vi "read PointGrey metadata file.vi"(0 "PointGrey metadata file path":path) -> (3 "Frames On File":i32, 4 "Created Csv File":path, 6 "Frame Drops":i64, 8 "Frames Acquired":i32, 10 "FrameCounter (processed)":i64[](array[numeric]), 13 "Separation Character":string, 15 "File Has Data":bool)   [LabVIEW 2010]
uses:
  <vilib>/Utility/file.llb/Read From Spreadsheet File (I64).vi
panel:
  out "Original File Lines":string[](array[string])
  out "Frequency (approximate)":ext format="%#.2g"
  out "PointGrey Timestamp (seconds)":ext[](array[numeric])
  out "TimeStamp (raw)":i64[](array[numeric])
  out "FrameCounter (raw)":i64[](array[numeric])
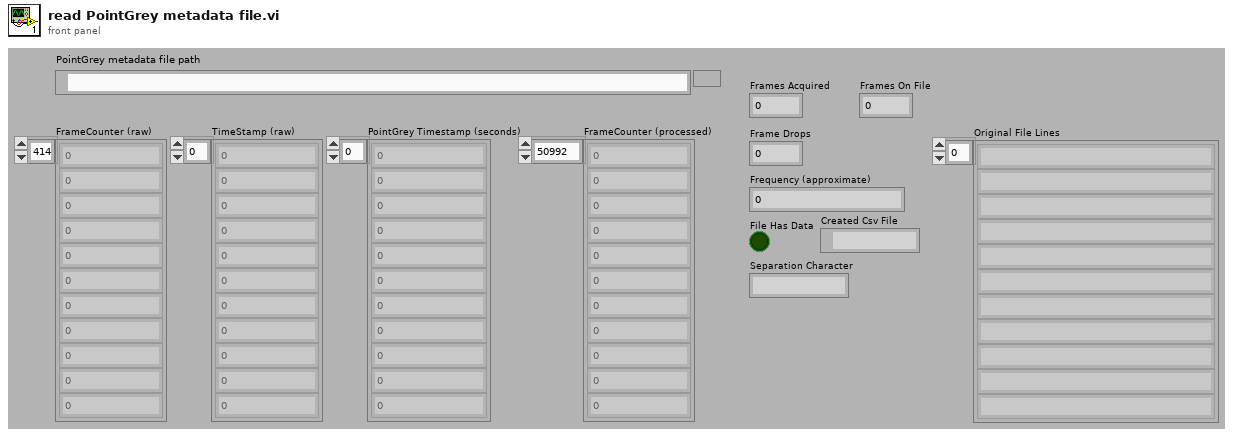
[diagram p1: front panel]
types:
  T1 = enum16{"open", "replace", "create", "open or create", "replace or create", "replace or create with confirmation"}
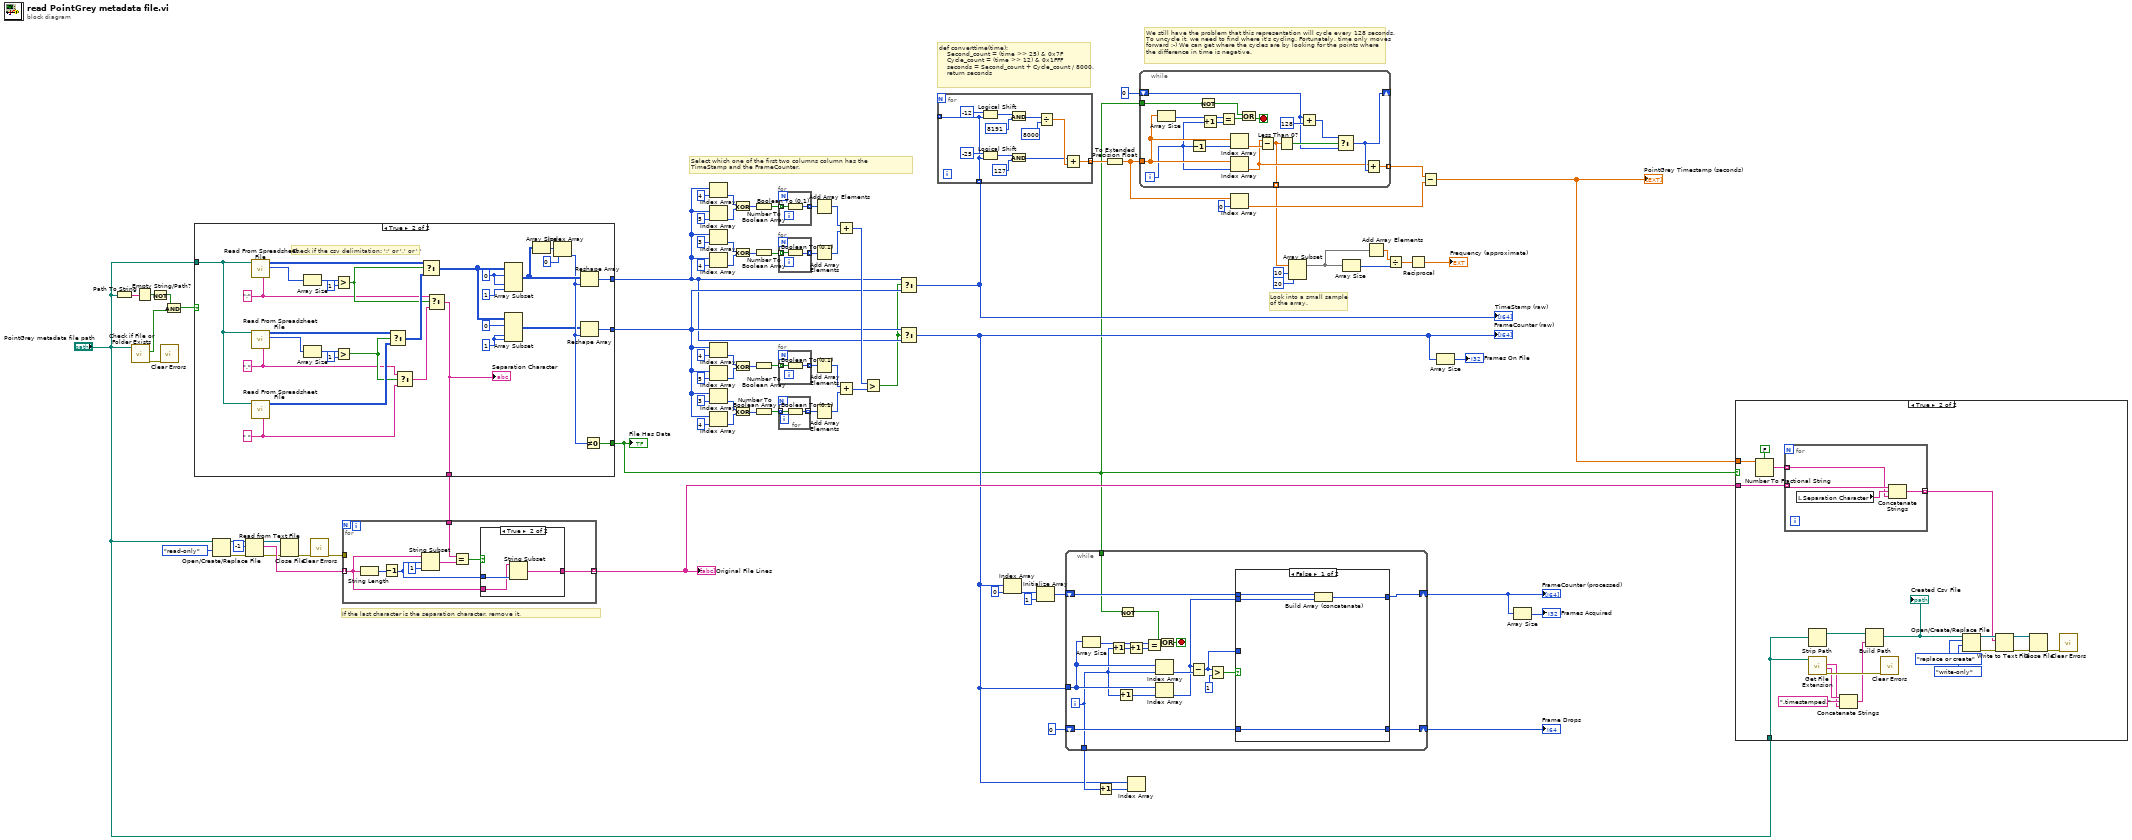
[diagram p0: block diagram]
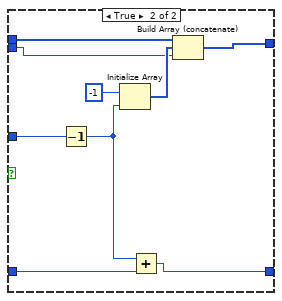
[diagram p4: hidden frame]
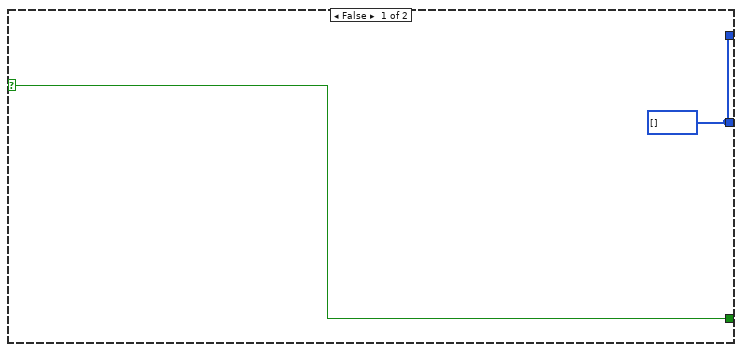
[diagram p5: hidden frame]
diagram:
  # "If the last character is the separation character, remove it."
  # "Select which one of the first two columns column has the\nTimeStamp and the FrameCounter."
  # "Look into a small sample\nof the array."
  # "We still have the problem that this representation will cycle every 128 seconds.\nTo uncycle it, we need to find where it's cycling. Fortunately, time only moves\nforward :-) We can get where the cycles are by looking for the points where\nthe difference in time is negative."
  # "def converttime(time):\n    Second_count = (time >> 25) & 0x7F\n    Cycle_count = (time >> 12) & 0x1FFF\n    seconds = Second_count + Cycle_count / 8000.\n    return seconds"
  n1 = Path To String(path="PointGrey metadata file path") -> (string=w5:string)
  n2 = call <vilib>:"Check if File or Folder Exists.vi"("path"="PointGrey metadata file path") -> ("error out"=w84:errorcluster, "file or folder exists?"=w83:bool)  [unwired: 8 in, 1 out]
  n3 = Empty String/Path?(string/path=w5) -> (empty?=w4:bool)
  n4 = Not(x=w4) -> (.not. x?=w2:bool)
  n5 = call <vilib>:"Clear Errors.vi"("error in (no error)"=w84) -> ()  [unwired: 6 in, 1 out]
  n6 = And(x=w2, y=w83) -> (x .and. y?=w3:bool)
  n7 = case shown="True" w3 {
    selector: w3 -> [w86 _]
    tunnel: "PointGrey metadata file path" -> [_ w108]
    tunnel: [w85 w101] -> w27
    tunnel: [w86 w109] -> w1
    tunnel: [w85 w99] -> w28
    tunnel: [_ w87] -> w16
    frame False {
      w85 = i64[] []
    }
    frame True {
      w89 = 1 ("length")
      w92 = " " ("delimiter (\\t)")
      w90 = 0 ("index")
      w93 = "," ("delimiter (\\t)")
      w95 = ";" ("delimiter (\\t)")
      # "Check if the csv delimitation: ';' or ',' or ' '"
      n8 = call-poly <vilib>:"Read From Spreadsheet File.vi"("delimiter (\\t)"=w95, "file path (dialog if empty)"=w108) -> ("first row"=w115:i64[], "all rows"=w114:i64[][])  [unwired: 5 in, 3 out]
      n9 = call-poly <vilib>:"Read From Spreadsheet File.vi"("delimiter (\\t)"=w93, "file path (dialog if empty)"=w108) -> ("first row"=w105:i64[], "all rows"=w104:i64[][])  [unwired: 5 in, 3 out]
      n10 = call-poly <vilib>:"Read From Spreadsheet File.vi"("delimiter (\\t)"=w92, "file path (dialog if empty)"=w108) -> ("all rows"=w103:i64[][])  [unwired: 5 in, 4 out]
      n11 = Array Size(array=w115) -> (size(s)=w117:i32)
      n12 = Array Size(array=w105) -> (size(s)=w106:i32)
      n13 = Greater?(x=w117, y=1) -> (0:w96:bool)
      n14 = Greater?(x=w106, y=1) -> (0:w94:bool)
      n15 = Select(t=w104, s=w94, f=w103) -> (s? t:f=w102:i64[][])
      n16 = Select(t=w93, s=w94, f=w92) -> (s? t:f=w91:string)
      n17 = Select(t=w114, s=w96, f=w102) -> (s? t:f=w88:i64[][])
      n18 = Select(t=w95, s=w96, f=w91) -> (s? t:f=w87:string)
      "Separation Character" <- w87
      n19 = Array Subset(array=w88, index (row)=w90, index (col)=w90, length (col)=1 ("length")) -> (w110:i64[][])  [unwired: 1 in]
      n20 = Array Subset(array=w88, index (row)=0 ("index"), index (col)=w89, length (col)=w89) -> (w97:i64[][])  [unwired: 1 in]
      n21 = Array Size(array=w110) -> (size(s)=w112:i32[])
      n22 = Index Array(array=w112, index=0) -> (element=w98:i32)
      n23 = Reshape Array(w110, w98) -> (w101:i64[])
      n24 = Reshape Array(w97, w98) -> (w99:i64[])
      n25 = Not Equal To 0?(x=w98) -> (x != 0?=w109:bool)
    }
  }
  "File Has Data" <- w1
  n26 = Open/Create/Replace File(file path (use dialog)="PointGrey metadata file path", access (0:read/write)=enum16{"read/write", "read-only", "write-only"}."read-only") -> (refnum out=w23:refnum<file>, error out=w24:errorcluster)  [unwired: 4 in, 1 out]
  n27 = Read from Text File(file (use dialog)=w23, count=-1, error in=w24) -> (refnum out=w18:refnum<file>, text=w20:string[], error out=w19:errorcluster)  [unwired: 1 in, 1 out]
  n28 = Close File(refnum=w18, error in=w19) -> (error out=w17:errorcluster)  [unwired: 1 out]
  n29 = call <vilib>:"Clear Errors.vi"("error in (no error)"=w17) -> ("error out"=w14:errorcluster)  [unwired: 6 in]
  n30 = for {
    tunnel: w20 -> [w121] mode=indexing
    tunnel: w14 -> [_]
    tunnel: w16 -> [w122]
    tunnel: [w119] -> w12 mode=indexing
    n31 = String Length(string=w121) -> (length=w125:i32)
    n32 = Decrement(x=w125) -> (x-1=w120:i32)
    n33 = String Subset(string=w121, offset (0)=w120, length (rest)=1 ("length (rest)")) -> (substring=w123:string)
    n34 = Equal?(x=w122, y=w123) -> (x = y?=w118:bool)
    n35 = case shown="True" w118 {
      tunnel: w121 -> [w126 w127]
      tunnel: w120 -> [_ w129]
      tunnel: [w126 w128] -> w119
      frame False {
      }
      frame True {
        n36 = String Subset(string=w127, length (rest)=w129) -> (substring=w128:string)  [unwired: 1 in]
      }
    }
  }
  "Original File Lines" <- w12
  n37 = Index Array(array=w27, index=4) -> (element=w45:i64)
  n38 = Index Array(array=w27, index=5) -> (element=w44:i64)
  n39 = Index Array(array=w27, index=3) -> (element=w59:i64)
  n40 = Index Array(array=w27, index=4) -> (element=w60:i64)
  n41 = Index Array(array=w28, index=4) -> (element=w58:i64)
  n42 = Index Array(array=w28, index=5) -> (element=w57:i64)
  n43 = Index Array(array=w28, index=3) -> (element=w36:i64)
  n44 = Index Array(array=w28, index=4) -> (element=w37:i64)
  n45 = Exclusive Or(1:w44, 2:w45) -> (0:w46:i64)
  n46 = Exclusive Or(1:w60, 2:w59) -> (0:w54:i64)
  n47 = Exclusive Or(1:w57, 2:w58) -> (0:w53:i64)
  n48 = Exclusive Or(1:w37, 2:w36) -> (0:w40:i64)
  n49 = Number To Boolean Array(number=w46) -> (Boolean array=w47:bool[])
  n50 = Number To Boolean Array(number=w54) -> (Boolean array=w52:bool[])
  n51 = Number To Boolean Array(number=w53) -> (Boolean array=w49:bool[])
  n52 = Number To Boolean Array(number=w40) -> (Boolean array=w41:bool[])
  n53 = for {
    tunnel: w41 -> [w131] mode=indexing
    tunnel: [w130] -> _ mode=indexing
    tunnel: [w130] -> w15 mode=indexing
    n54 = Boolean To (0,1)(Boolean=w131) -> (0, 1=w130:i16)
  }
  n55 = for {
    tunnel: w47 -> [w133] mode=indexing
    tunnel: [w132] -> w48 mode=indexing
    n56 = Boolean To (0,1)(Boolean=w133) -> (0, 1=w132:i16)
  }
  n57 = for {
    tunnel: w52 -> [w135] mode=indexing
    tunnel: [w134] -> w51 mode=indexing
    n58 = Boolean To (0,1)(Boolean=w135) -> (0, 1=w134:i16)
  }
  n59 = for {
    tunnel: w49 -> [w137] mode=indexing
    tunnel: [w136] -> w50 mode=indexing
    n60 = Boolean To (0,1)(Boolean=w137) -> (0, 1=w136:i16)
  }
  n61 = Add Array Elements(numeric array=w48) -> (sum=w34:i16)
  n62 = Add Array Elements(numeric array=w51) -> (sum=w35:i16)
  n63 = Add Array Elements(numeric array=w50) -> (sum=w33:i16)
  n64 = Add Array Elements(numeric array=w15) -> (sum=w32:i16)
  n65 = Add(x=w34, y=w35) -> (x+y=w30:i16)
  n66 = Add(x=w33, y=w32) -> (x+y=w31:i16)
  n67 = Greater?(x=w30, y=w31) -> (0:w26:bool)
  n68 = Select(t=w27, s=w26, f=w28) -> (s? t:f=w29:i64[])
  "TimeStamp (raw)" <- w29
  n69 = Select(t=w28, s=w26, f=w27) -> (s? t:f=w7:i64[])
  "FrameCounter (raw)" <- w7
  n70 = for {
    tunnel: [w139] -> _ mode=indexing
    tunnel: [w140] -> w82 mode=indexing
    tunnel: w29 -> [w139] mode=indexing
    n71 = Logical Shift(y=i8 -12, x=w139) -> (x << y=w148:i64)
    n72 = Logical Shift(y=i8 -25, x=w139) -> (x << y=w145:i64)
    n73 = And(x=w148, y=i64 8191) -> (x .and. y?=w143:i64)
    n74 = And(x=w145, y=i64 127) -> (x .and. y?=w138:i64)
    n75 = Divide(x=w143, y=i64 8000) -> (x/y=w141:dbl)
    n76 = Add(x=w138, y=w141) -> (x+y=w140:dbl)
  }
  n77 = Index Array(array=w7, index=0) -> (element=w68:i64)
  n78 = Initialize Array(w68, 1 ("dimension size")) -> (w66:i64[])
  n79 = while {
    tunnel: w7 -> [w166]
    shift-right: [w158] -> w9
    shift-left: w66 -> [w160]
    shift-right: [w157] -> w64
    shift-left: i64 0 ("y") -> [w156]
    tunnel: [w154] -> w11
    tunnel: w1 -> [w151]
    i -> [w154]
    stop <- w152 stop-if-true
    n80 = Array Size(array=w166) -> (size(s)=w168:i32)
    n81 = Increment(x=w154) -> (x+1=w153:i32)
    n82 = Increment(x=w154) -> (x+1=w163:i32)
    n83 = Not(x=w151) -> (.not. x?=w150:bool)
    n84 = Increment(x=w153) -> (x+1=w164:i32)
    n85 = Equal?(x=w168, y=w164) -> (x = y?=w167:bool)
    n86 = Index Array(array=w166, index=w154) -> (element=w165:i64)
    n87 = Index Array(array=w166, index=w163) -> (element=w159:i64)
    n88 = Or(x=w150, y=w167) -> (x .or. y?=w152:bool)
    n89 = Subtract(x=w159, y=w165) -> (x-y=w155:i64)
    n90 = Greater?(x=w155, y=i64 1) -> (0:w161:bool)
    n91 = case shown="False" w161 {
      tunnel: w160 -> [w172 w176]
      tunnel: w159 -> [w171 w173]
      tunnel: [w170 w175] -> w158
      tunnel: [w169 w180] -> w157
      tunnel: w156 -> [w169 w181]
      tunnel: w155 -> [_ w178]
      frame False {
        n92 = Build Array (concatenate)(w172, w171) -> (w170:i64[])
      }
      frame True {
        n93 = Decrement(x=w178) -> (x-1=w174:i64)
        n94 = Initialize Array(i64 -1 ("element"), w174) -> (w177:i64[])
        n95 = Add(x=w174, y=w181) -> (x+y=w180:i64)
        n96 = Build Array (concatenate)(w176, w177, w173) -> (w175:i64[])
      }
    }
  }
  "Frame Drops" <- w64
  "FrameCounter (processed)" <- w9
  n97 = Increment(x=w11) -> (x+1=w10:i32)
  n98 = To Extended Precision Float(1:w82) -> (0:w76:ext[])
  n99 = Index Array(array=w7, index=w10) -> ()  [unwired: 1 out]
  n100 = while {
    tunnel: w76 -> [w197]
    shift-right: [w191] -> _
    shift-left: i64 0 ("y") -> [w193]
    tunnel: [w190] -> w80 mode=indexing
    tunnel: [w185] -> w73 mode=indexing
    tunnel: w1 -> [w183]
    i -> [w187]
    stop <- w184 stop-if-true
    n101 = Array Size(array=w197) -> (size(s)=w199:i32)
    n102 = Decrement(x=w187) -> (x-1=w188:i32)
    n103 = Not(x=w183) -> (.not. x?=w182:bool)
    n104 = Increment(x=w187) -> (x+1=w186:i32)
    n105 = Equal?(x=w199, y=w186) -> (x = y?=w198:bool)
    n106 = Index Array(array=w197, index=w188) -> (element=w192:ext)
    n107 = Index Array(array=w197, index=w187) -> (element=w189:ext)
    n108 = Or(x=w182, y=w198) -> (x .or. y?=w184:bool)
    n109 = Subtract(x=w189, y=w192) -> (x-y=w185:ext)
    n110 = Less Than 0?(x=w185) -> (x < 0?=w196:bool)
    n111 = Add(x=w193, y=i64 128) -> (x+y=w195:i64)
    n112 = Select(t=w195, s=w196, f=w193) -> (s? t:f=w191:i64)
    n113 = Add(x=w189, y=w191) -> (x+y=w190:ext)
  }
  n114 = Index Array(array=w76, index=0) -> (element=w79:ext)
  n115 = Array Subset(array=w73, index=10, length=20) -> (w71:ext[])
  n116 = Array Size(array=w71) -> (size(s)=w75:i32)
  n117 = Add Array Elements(numeric array=w71) -> (sum=w77:ext)
  n118 = Divide(x=w77, y=w75) -> (x/y=w74:ext)
  n119 = Reciprocal(x=w74) -> (1/x=→"Frequency (approximate)":ext)
  n120 = Subtract(x=w80, y=w79) -> (x-y=w13:ext[])
  "PointGrey Timestamp (seconds)" <- w13
  n121 = Array Size(array=w7) -> (size(s)=→"Frames On File":i32)
  n122 = Array Size(array=w9) -> (size(s)=→"Frames Acquired":i32)
  n123 = case shown="True" w1 {
    tunnel: w13 -> [_ w219]
    tunnel: w12 -> [_ w218]
    tunnel: "PointGrey metadata file path" -> [_ w209]
    frame False {
    }
    frame True {
      n124 = Number To Fractional String(use system decimal point (T)=FALSE, number=w219) -> (F-format string=w217:string[])  [unwired: 2 in]
      n125 = for {
        tunnel: w218 -> [w223] mode=indexing
        tunnel: w217 -> [w221] mode=indexing
        tunnel: [w220] -> w210 mode=indexing
        n126 = local read "Separation Character"() -> (w222:string)
        n127 = Concatenate Strings(w223, w222, w221) -> (w220:string)
      }
      n128 = Strip Path(path=w209) -> (stripped path=w204:path)  [unwired: 1 out]
      n129 = call <vilib>:"Get File Extension.vi"("file"=w209) -> ("error out"=w208:errorcluster, "filename without extension"=w207:string, "lowercase file extension"=w205:string)  [unwired: 7 in, 1 out]
      n130 = Concatenate Strings(w207, ".timestamped." ("string"), w205) -> (w203:string)
      n131 = Build Path(base path=w204, name or relative path=w203) -> (appended path=w202:path)
      "Created Csv File" <- w202
      n132 = call <vilib>:"Clear Errors.vi"("error in (no error)"=w208) -> ()  [unwired: 6 in, 1 out]
      n133 = Open/Create/Replace File(file path (use dialog)=w202, operation (0:open)=T1."replace or create", access (0:read/write)=enum16{"read/write", "read-only", "write-only"}."write-only") -> (refnum out=w212:refnum<file>, error out=w211:errorcluster)  [unwired: 3 in, 1 out]
      n134 = Write to Text File(file (use dialog)=w212, text=w210, error in=w211) -> (refnum out=w215:refnum<file>, error out=w214:errorcluster)  [unwired: 1 in, 1 out]
      n135 = Close File(refnum=w215, error in=w214) -> (error out=w216:errorcluster)  [unwired: 1 out]
      n136 = call <vilib>:"Clear Errors.vi"("error in (no error)"=w216) -> ()  [unwired: 6 in, 1 out]
    }
  }
